vi "Time.vi"() -> (3 "Timestamp":string)   [LabVIEW 2024]
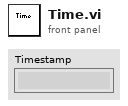
[diagram p1: front panel]
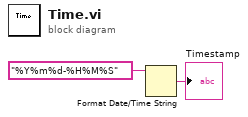
[diagram p0: block diagram]
diagram:
  n1 = Format Date/Time String(time format string (%c)="%Y%m%d-%H%M%S") -> (date/time string=→"Timestamp":string)  [unwired: 2 in]
